vi "test.vi"() -> ()   [LabVIEW 2019]
uses:
  <vilib>/Platform/TimedLoop/XDataNode/timing_clust.ctl
  <vilib>/Platform/TimedLoop/XDataNode/nitl_modes.ctl
  <vilib>/Platform/TimedLoop/XDataNode/wakeup.ctl
  <vilib>/platform/TimedLoop/XDataNode/XDataNode.xnode
  <vilib>/Platform/TimedLoop/XDataNode/XDNodeRunTimeDep.lvlib
  KNRm_ReMi_OS6_436Motor.lvlibp
panel:
  in  "Port":enum16{"SM1(S1&S2)", "SM2(S3&S4)", "SM3(S5&S6)"}(ring)
  out "PulseCounter+/-":i32
  out "motordegree":dbl=0.5
  in  "stop":bool
  in  "vel(deg/sec)":dbl
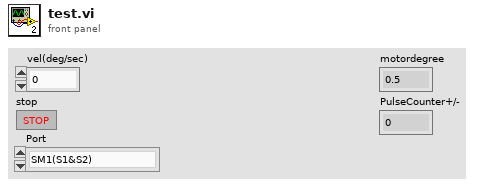
[diagram p1: front panel]
types:
  T1 = typedef "XDNodeRunTimeDep.lvlib/timing_clust.ctl" = cluster{"Expected End [f-1]":u64, "Actual End [f-1]":u64, "Finished Late? [f-1]":bool, "Expected End [i-1]":u64, "Actual End [i-1]":u64, "Finished Late? [i-1]":bool, "Expected Start [i]":u64, "Actual Start [i]":u64, "Expected Start [f]":u64, "Actual Start [f]":u64, "Source Name":string, "Structure Name":string, "Period":i64, "Deadline":i64, "Offset":i64, "Start":i64, "Priority":i32, "Timeout":i32, "Mode":T2, "Wakeup Reason":T3, "Error":errorcluster, "Source Type":string, "Secondary Source Type":string, "Global End Time":u64, "Global Start Time":u64, "Frame Duration":u64, "Iteration Duration":u64, "Assigned CPU":i32, "I/O Scan Engine Mode":u32}
  T2 = typedef "XDNodeRunTimeDep.lvlib/nitl_modes.ctl" = enum32{"No Change", "Process missed periods, maintain original phase", "Discard missed periods, maintain original phase", "Process missed periods, ignore original phase", "Discard missed periods, ignore original phase"}
  T3 = typedef "XDNodeRunTimeDep.lvlib/wakeup.ctl" = enum32{"Normal", "Aborted", "Asynchronous wakeup", "Timing source error", "Timed loop error", "Timeout"}
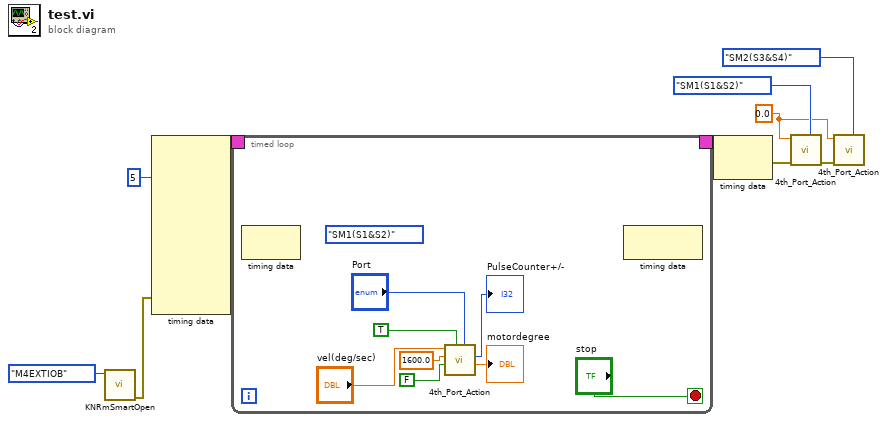
[diagram p0: block diagram]
diagram:
  w3 = 0.0 ("vel(deg/sec)")
  n1 = call "KNRmSmartOpen.vi"("INI FPGA MODE"=enum16{"Original", "M4EXTIOB"}."M4EXTIOB") -> ("error out"=w1:errorcluster)  [unwired: 7 in, 3 out]
  n2 = node-c288(i64 5 ("Period"), w1) -> (w10:T1)  [unwired: 8 in]
  n3 = timed-loop {
    timing: w10 -> [_]
    timing-out: [_] -> w9
    stop <- "stop" stop-if-true
    (unwired) enum16{"SM1(S1&S2)", "SM2(S3&S4)", "SM3(S5&S6)"}."SM1(S1&S2)" ("Port")
    n4 = node-c288() -> ()  [unwired: 1 in, 1 out]
    n5 = call "4th_Port_Action.vi"("Port"="Port", "EN"=TRUE, "ResetCounter"=FALSE ("Enable"), "step"=1600.0, "vel(deg/sec)"="vel(deg/sec)") -> ("motordegree"=→"motordegree":dbl, "PulseCounter+/-"=→"PulseCounter+/-":i32)  [unwired: 4 in, 1 out]
    n6 = node-c288() -> ()  [unwired: 1 in, 1 out]
  }
  n7 = node-c288(w9) -> (w7:errorcluster)
  n8 = call "4th_Port_Action.vi"("Port"=enum16{"SM1(S1&S2)", "SM2(S3&S4)", "SM3(S5&S6)"}."SM1(S1&S2)", "error in"=w7, "vel(deg/sec)"=w3) -> ("error out"=w5:errorcluster)  [unwired: 6 in, 2 out]
  n9 = call "4th_Port_Action.vi"("Port"=enum16{"SM1(S1&S2)", "SM2(S3&S4)", "SM3(S5&S6)"}."SM2(S3&S4)", "error in"=w5, "vel(deg/sec)"=w3) -> ()  [unwired: 6 in, 3 out]
